vi "onSelfStop.vi"(11 "SMO":refnum<class "SMO.lvclass">) -> ()   [LabVIEW 2013, in "SMO.lvclass"]
uses:
  SMO.lvclass
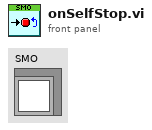
[diagram p1: front panel]
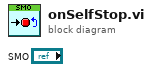
[diagram p0: block diagram]
diagram:
